vi "PH_Beckhoff_PP_Control.set PSDB Stuff.vi"(0 "i ref in":refnum<vi>, 5 "error in":errorcluster) -> (14 "i ref out":refnum<vi>, 19 "error out":errorcluster)   [LabVIEW 2014]
doc: "Within this VI several attributes concerning the PSDB are set."
uses:
  PH_Beckhoff_PP_Control.lvlib
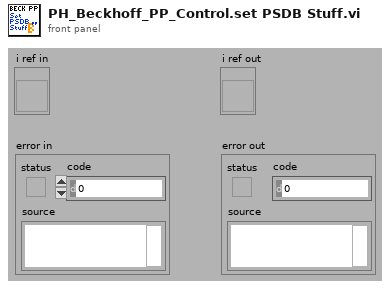
[diagram p1: front panel]
types:
  T1 = typedef "Data_Status.ctl" = i16
  T2 = typedef "PHELIX-Subsystems.ctl" = i32
  T3 = typedef "PH_Beckhoff_PP_Control.lvlib/PH_Beckhoff_PP_Control.i attribute.ctl" = cluster{"PP Conductivity Control":cluster{"PSDB":cluster{"Status Service ID":i32, "Instance ID":i32, "Data Status":T1, "Ref Status":refnum<vi>, "Error Code":i32}, "Status":cluster{"GUI Ref":refnum<vi>, "Status Service ID":i32, "Status":T4}, "DIs":cluster{"Device on":cluster{"GUI Ref":refnum<vi>, "# in Data":i32}, "Conductivity ok":cluster{"GUI Ref":refnum<vi>, "# in Data":i32}, "Temperature ok":cluster{"GUI Ref":refnum<vi>, "# in Data":i32}, "Alarm":cluster{"GUI Ref":refnum<vi>, "# in Data":i32}}, "PSDB Thread":cluster{"Ref":refnum<vi>, "Q-Ref":refnum<queue>}}, "PP Mercury Control":cluster{"PSDB":cluster{"Status Service ID":i32, "Instance ID":i32, "Data Status":T1, "Ref Status":refnum<vi>, "Error Code":i32}, "Status":cluster{"GUI Ref":refnum<vi>, "Status Service ID":i32, "Status":T4}, "on since:":cluster{"GUI Ref":refnum<vi>, "Service ID":i32, "Time":string}, "DIs":cluster{"Device on":cluster{"GUI Ref":refnum<vi>, "# in Data":i32}, "Alarm":cluster{"GUI Ref":refnum<vi>, "# in Data":i32}}, "AIs":cluster{"Concentration":cluster{"GUI Ref":refnum<vi>, "# in Data":i32}}, "PSDB Thread":cluster{"Ref":refnum<vi>, "Q-Ref":refnum<queue>}}, "PSDB":cluster{"Shot #":i32, "Subsystem":T2, "Controller":string, "Data Source":string, "Password":string}, "Handle GUI Refs Attributes":T5}
  T4 = typedef "Status.ctl" = i16
  T5 = typedef "PH Handle GUI Refs.Attributes.ctl" = cluster{"Event":refnum<user-event>, "Event registered":refnum<k4>, "GUI Refs stored":refnum<k4>}
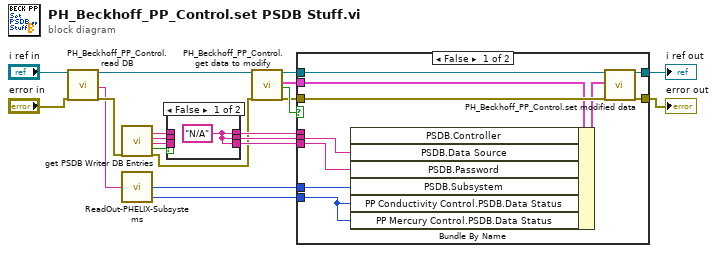
[diagram p0: block diagram]
diagram:
  n1 = call "PH_Beckhoff_PP_Control.read DB.vi"("i ref in"="i ref in", "error in (no error)"="error in") -> ("i ref out"=w5:refnum<vi>, "PSDB Instance Information: Subsystem"=w9:string, "error out"=w12:errorcluster)  [unwired: 13 in, 2 out]
  n2 = call "get PSDB Writer DB Entries.vi"("error in"=w12) -> ("PSDB Controller"=w15:string, "PSDB Data Source"=w17:string, "PSDB Password"=w19:string, "all information available?"=w13:bool, "error out"=w14:errorcluster)  [unwired: 14 in]
  n3 = call "ReadOut-PHELIX-Subsystems.vi"("Config DB Subsystem"=w9) -> ("Metadata.Data Status"=w11:T1, "Metadata.Subsystem"=w10:T2)  [unwired: 2 in, 1 out]
  n4 = case shown="False" w13 {
    tunnel: w15 -> [_ w25]
    tunnel: [w22 w25] -> w16
    tunnel: w17 -> [_ w24]
    tunnel: [w22 w24] -> w18
    tunnel: [w22 w23] -> w20
    tunnel: w19 -> [_ w23]
    frame False {
      w22 = "N/A" ("PSDB Controller")
    }
    frame True {
    }
  }
  n5 = call "PH_Beckhoff_PP_Control.get data to modify.vi"("i ref in"=w5, "error in (no error)"=w14) -> ("i ref out"=w6:refnum<vi>, "i attribute"=w7:T3, "timed out"=w8:bool, "error out"=w2:errorcluster)  [unwired: 14 in]
  n6 = case shown="False" w8 {
    tunnel: w2 -> [w36 w37]
    tunnel: [w35 w37] -> w3
    tunnel: w6 -> [w34 w38]
    tunnel: [w33 w38] -> w21
    tunnel: w7 -> [w32 _]
    tunnel: w10 -> [w30 _]
    tunnel: w11 -> [w29 _]
    tunnel: w16 -> [_ _]
    tunnel: w18 -> [w27 _]
    tunnel: w20 -> [w26 _]
    frame False {
      n7 = Bundle By Name(cluster=w32, "PSDB.Data Source"=w27, "PSDB.Password"=w26, "PSDB.Subsystem"=w30, "PP Conductivity Control.PSDB.Data Status"=w29, "PP Mercury Control.PSDB.Data Status"=w29) -> (w31:T3, "PSDB.Controller"=w28:string)
      n8 = call "PH_Beckhoff_PP_Control.set modified data.vi"("i ref in"=w34, "i attribute"=w31, "error in (no error)"=w36) -> ("i ref out"=w33:refnum<vi>, "error out"=w35:errorcluster)  [unwired: 15 in]
    }
    frame True {
    }
  }
  "i ref out" <- w21
  "error out" <- w3
